vi "test Sort by Priority.vi"(8 "error in (no error)":errorcluster, 11 "TestCase in":refnum<class "Configuration Tests.lvclass">) -> (0 "error out":errorcluster, 3 "TestCase out":refnum<class "Configuration Tests.lvclass">)   [LabVIEW 2017, in "Configuration Tests.lvclass"]
uses:
  Configuration Tests.lvclass
  Mock Classes/Transfer Group/Mock Transfer Group.lvclass
  C:/github/data-sharing-framework/Data Sharing Framework Core/Engine/Classes/Transfer Group/Transfer Group.lvclass
  Engine/Classes/Transfer Group/Transfer Group.lvclass/Transfer Group.ctl
  Engine/Classes/Timing/Timing.lvclass/Timing.ctl
  <vilib>/addons/_JKI Toolkits/VI Tester/TestCase.llb/TestCase.lvclass
  Engine/Classes/Transfer Group/Transfer Group.lvclass
  Engine/Classes/Timing/Timing.lvclass
  C:/Program Files (x86)/National Instruments/LabVIEW 2017/vi.lib/addons/_JKI Toolkits/VI Tester/TestCase.llb/TestCase.lvclass
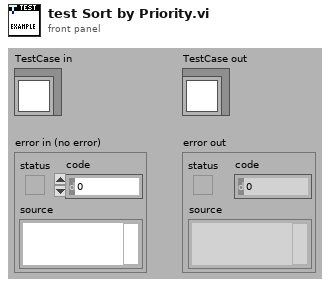
[diagram p1: front panel]
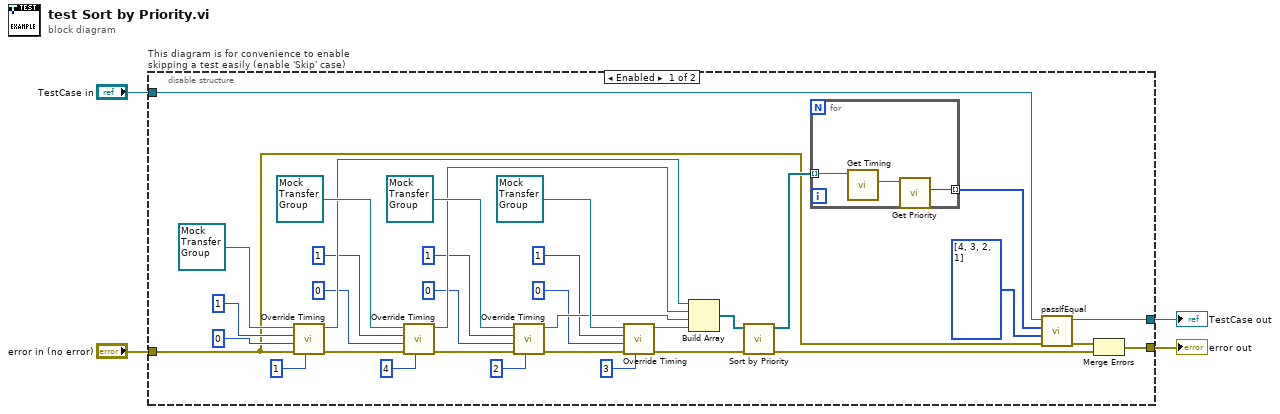
[diagram p0: block diagram]
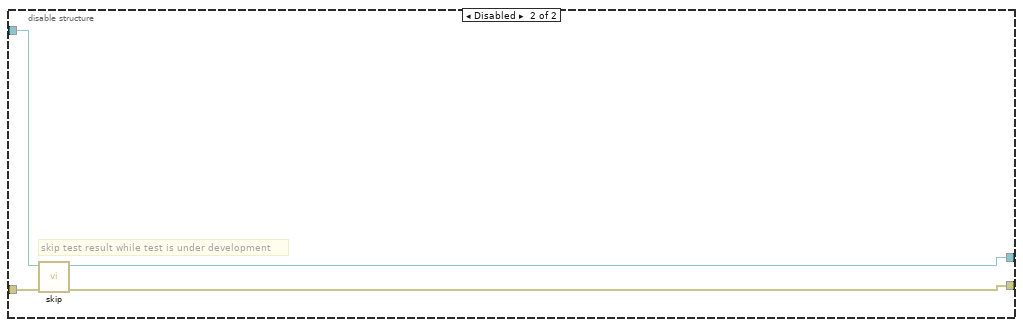
[diagram p2: hidden frame]
diagram:
  n1 = disable-structure "This diagram is for convenience to enable skipping a test easily (enable 'Skip' case)" shown="Enabled" {
    disable-tunnel: "TestCase in" -> [w25 w45]
    disable-tunnel: [w23 w43] -> w1
    disable-tunnel: [w6 w44] -> w3
    disable-tunnel: "error in (no error)" -> [w7 w42]
    frame Enabled {
      n2 = call "Override Timing.vi"("Priority"=u64 1, "error in (no error)"=w7, "Offset"=u64 0, "Decimation"=u64 1, "Mock Transfer Group in"=refnum<class "Mock Transfer Group.lvclass"> refnum) -> ("error out"=w34:errorcluster, "Mock Transfer Group out"=w30:refnum<class "Mock Transfer Group.lvclass">)  [unwired: 5 in]
      n3 = call "Override Timing.vi"("Priority"=u64 4, "error in (no error)"=w34, "Offset"=u64 0, "Decimation"=u64 1, "Mock Transfer Group in"=refnum<class "Mock Transfer Group.lvclass"> refnum) -> ("error out"=w33:errorcluster, "Mock Transfer Group out"=w29:refnum<class "Mock Transfer Group.lvclass">)  [unwired: 5 in]
      n4 = call "Override Timing.vi"("Priority"=u64 2, "error in (no error)"=w33, "Offset"=u64 0, "Decimation"=u64 1, "Mock Transfer Group in"=refnum<class "Mock Transfer Group.lvclass"> refnum) -> ("error out"=w32:errorcluster, "Mock Transfer Group out"=w28:refnum<class "Mock Transfer Group.lvclass">)  [unwired: 5 in]
      n5 = call "Override Timing.vi"("Priority"=u64 3, "error in (no error)"=w32, "Offset"=u64 0, "Decimation"=u64 1, "Mock Transfer Group in"=refnum<class "Mock Transfer Group.lvclass"> refnum) -> ("error out"=w31:errorcluster, "Mock Transfer Group out"=w27:refnum<class "Mock Transfer Group.lvclass">)  [unwired: 5 in]
      n6 = Build Array(w30, w29, w28, w27) -> (w26:refnum<class "Mock Transfer Group.lvclass">[])
      n7 = call "Sort by Priority.vi"("error in (no error)"=w31, "Transfer Groups"=w26) -> ("error out"=w5:errorcluster, "sorted Transfer Groups"=w22:refnum<class "Transfer Group.lvclass">[])  [unwired: 8 in]
      n8 = for {
        tunnel: w22 -> [w41] mode=indexing
        tunnel: [w39] -> w21 mode=indexing
        n9 = call "Get Timing.vi"("Transfer Group in"=w41) -> ("Timing"=w40:refnum<class "Timing.lvclass">)  [unwired: 9 in, 1 out]
        n10 = call "Get Priority.vi"("Timing in"=w40) -> ("Priority"=w39:u64)  [unwired: 9 in, 1 out]
      }
      n11 = call-dynamic "passIfEqual.vi"("error in (no error)"=w7, "y"=u64[] [4, 3, 2, 1], "x"=w21, "TestCase in"=w25) -> ("error out"=w24:errorcluster, "TestCase out"=w23:refnum<class "Configuration Tests.lvclass">)  [unwired: 6 in]
      n12 = Merge Errors(w24, w5) -> (w6:errorcluster)
    }
    frame Disabled {
      # "skip test result while test is under development"
      n13 = call <vilib>:"skip.vi"("error in (no error)"=w42, "TestCase in"=w45) -> ("error out"=w44:errorcluster, "TestCase out"=w43:refnum<class "Configuration Tests.lvclass">)  [unwired: 8 in]
    }
  }
  "error out" <- w3
  "TestCase out" <- w1
